vi "Write Sequence Element Configuration.vi"(8 "error in (no error)":errorcluster, 10 "Configuration":T1 {"Duration" format="%#_6ps"}, 11 "Sequence Element in":refnum<class "Sequence Element.lvclass">) -> (0 "error out":errorcluster, 3 "Sequence Element out":refnum<class "Sequence Element.lvclass">)   [LabVIEW 2016, in "Sequence Element.lvclass"]
uses:
  Sequence Element.lvclass
  C:/github/LabActor/Template Module/Template Module.lvclass
  Sequence Element Configuration.ctl
  Template Module/Template Module.lvclass/Template Module.ctl
  Template Module/Write Configuration.vi
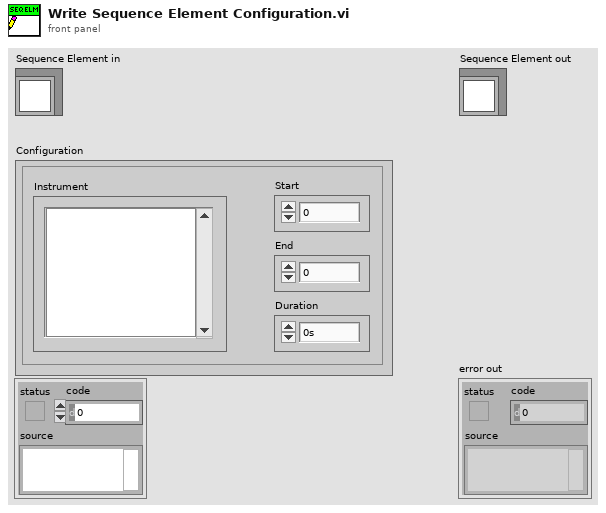
[diagram p1: front panel]
types:
  T1 = typedef "Sequence Element Configuration.ctl" = cluster{"Start":dbl, "End":dbl, "Duration":dbl, "Instrument":i32}
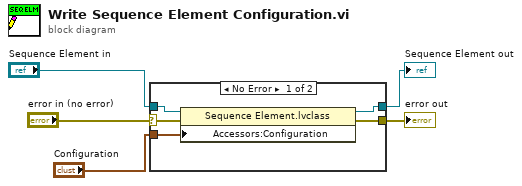
[diagram p0: block diagram]
diagram:
  n1 = case shown="No Error" "error in (no error)" {
    selector: "error in (no error)" -> [w7 w11]
    tunnel: [w6 w11] -> w4
    tunnel: [w8 w12] -> w2
    tunnel: "Sequence Element in" -> [w10 w12]
    tunnel: "Configuration" -> [w9 _]
    frame No Error {
      n2 = property class="Sequence Element.lvclass"(reference=w10, error in=w7, "Accessors:Configuration"=w9) -> (reference out=w8:refnum<class "Sequence Element.lvclass">, error out=w6:errorcluster)
    }
    frame Error {
    }
  }
  "error out" <- w4
  "Sequence Element out" <- w2
